vi "Day 2.1 - Score game.vi"(11 "input":string[](array[string])) -> (3 "output":u64)   [LabVIEW 2021]
panel:
  out "Array 2":i32[](array[numeric])
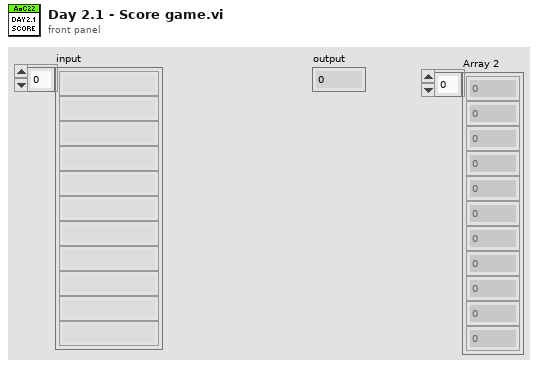
[diagram p1: front panel]
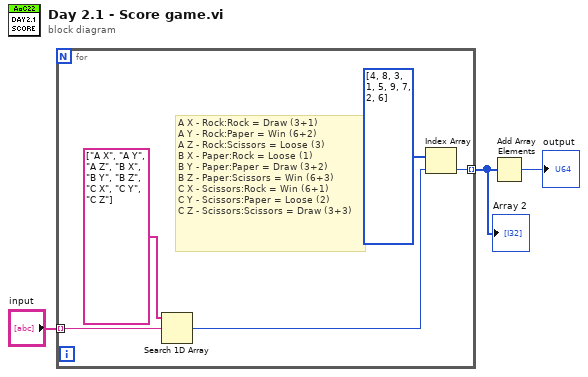
[diagram p0: block diagram]
diagram:
  n1 = for {
    tunnel: "input" -> [w8] mode=indexing
    tunnel: [w4] -> w3 mode=indexing
    # "A X - Rock:Rock = Draw (3+1)\nA Y - Rock:Paper = Win (6+2)\nA Z - Rock:Scissors = Loose (3)\nB X - Paper:Rock = Loose (1)\nB Y - Paper:Paper = Draw (3+2)\nB Z - Paper:Scissors = Win (6+3)\nC X - Scissors:Rock = Win (6+1)\nC Y - Scissors:Paper = Loose (2)\nC Z - Scissors:Scissors = Draw (3+3)"
    n2 = Search 1D Array(1D array=string[] ["A X", "A Y", "A Z", "B X", "B Y", "B Z", "C X", "C Y", "C Z"], element=w8) -> (index of element=w5:i32)  [unwired: 1 in]
    n3 = Index Array(array=i32[] [4, 8, 3, 1, 5, 9, 7, 2, 6], index=w5) -> (element=w4:i32)
  }
  "Array 2" <- w3
  n4 = Add Array Elements(numeric array=w3) -> (sum=→"output":i32)
